vi "svx_Colormap Area In.vi"(5 "Order":dbl, 7 "Range":T1, 11 "speed profile":cluster{"time [s]":dbl[], "speed [rpm]":dbl[]} {"speed [rpm]" format="%.2f"; "time [s]" format="%.2f"}) -> (0 "Order":dbl[](array[numeric]), 3 "Time(s)":dbl[](array[numeric]))   [LabVIEW 2017, in "SVX Colormap.xctl"]
uses:
  <vilib>/addons/_XControls/Colormap/SVX Colormap.xctl
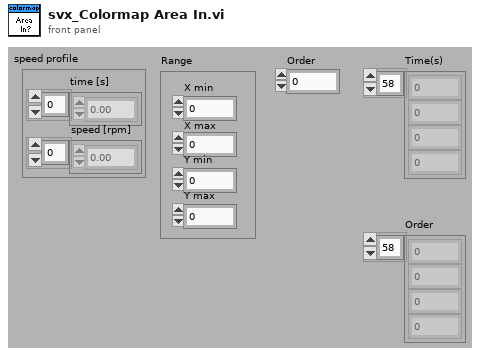
[diagram p1: front panel]
types:
  T1 = cluster{"X min":dbl, "X max":dbl, "Y min":dbl, "Y max":dbl}
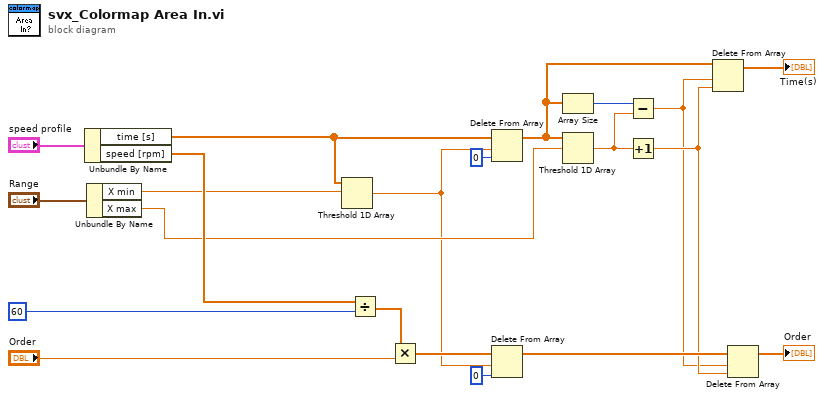
[diagram p0: block diagram]
diagram:
  n1 = Unbundle By Name("speed profile") -> ("time [s]"=w10:dbl[], "speed [rpm]"=w12:dbl[])
  n2 = Unbundle By Name("Range") -> ("X min"=w6:dbl, "X max"=w5:dbl)
  n3 = Threshold 1D Array(2:w6, 3:w10) -> (0:w3:dbl)  [unwired: 1 in]
  n4 = Divide(x=w12, y=60) -> (x/y=w9:dbl[])
  n5 = Multiply(x=w9, y="Order") -> (x*y=w7:dbl[])
  n6 = Delete From Array(array=w10, length=w3, index=0) -> (array with subset deleted=w14:dbl[])  [unwired: 1 out]
  n7 = Delete From Array(array=w7, length=w3, index=0) -> (array with subset deleted=w16:dbl[])  [unwired: 1 out]
  n8 = Array Size(array=w14) -> (size(s)=w19:i32)
  n9 = Threshold 1D Array(2:w5, 3:w14) -> (0:w18:dbl)  [unwired: 1 in]
  n10 = Subtract(x=w19, y=w18) -> (x-y=w13:dbl)
  n11 = Increment(x=w18) -> (x+1=w15:dbl)
  n12 = Delete From Array(array=w14, length=w13, index=w15) -> (array with subset deleted=→"Time(s)":dbl[])  [unwired: 1 out]
  n13 = Delete From Array(array=w16, length=w13, index=w15) -> (array with subset deleted=→"Order":dbl[])  [unwired: 1 out]
